vi "HDF5_Init_Validity_Refs.vi"(5 "HDF5 file ref":T2 format="%.0x", 9 "File Exists?":bool, 11 "error in":errorcluster) -> (4 "AlarmFileRefs":T1 {"Alarm_Source_dset" format="%.0x"; "Time_AlarmChange_dset" format="%.0x"; "Time_Valid_dset" format="%.0x"; "Alarm_Valid_dset" format="%.0x"; "Saturat_dset" format="%.0x"; "Group_ref" format="%.0x"; "Weath_Valid_dset" format="%.0x"; "Disdr_Valid_dset" format="%.0x"}, 15 "error out":errorcluster)   [LabVIEW 2018]
doc: "Set up the HDF5 data structure and initialize the references for the Noise1, Noise2, Noise3, and Noise4 Datasets (tables).\n\nData structure:\nNoise1 (Dataset) - 1024 element Double array (waveform) \nNoise2 (Dataset) - 1024 element Double array (waveform) \nNoise3 (Dataset) - 1024 element Double array (waveform) \nNoise4 (Dataset) - 1024 element Double array (waveform)"
uses:
  <vilib>/addons/h5labview2/base/hid_t.ctl
  HDF5_Validty_refs.ctl
  <vilib>/addons/h5labview2/base/lib_path.vi
  <vilib>/addons/h5labview2/base/H5Equery.vi
  lib_path_mod_20200519.vi
  <vilib>/addons/h5labview2/attrib/H5Awrite.llb/H5Awrite.xnode
  <vilib>/addons/h5labview2/group/H5G.lvlib
  <vilib>/addons/h5labview2/dataset/H5D.lvlib
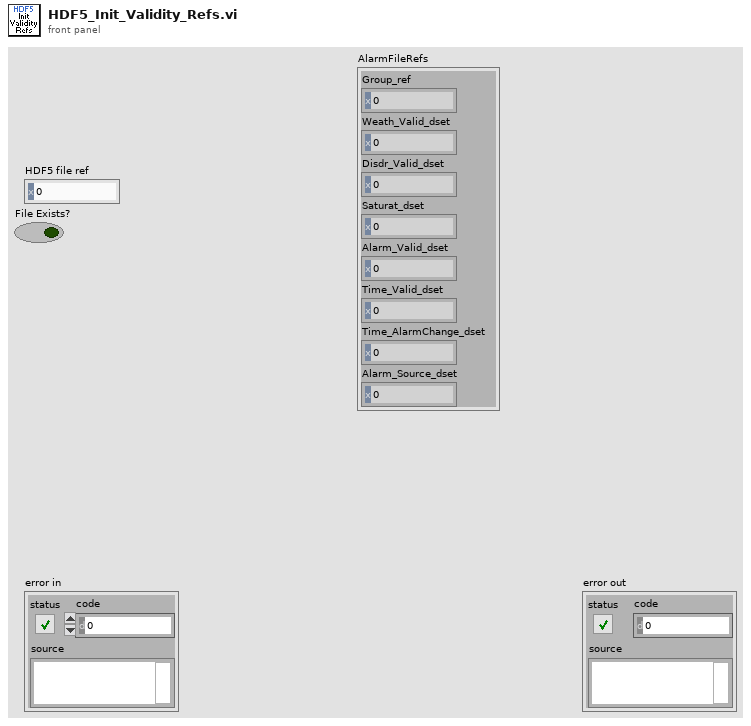
[diagram p1: front panel]
types:
  T1 = typedef "HDF5_Validty_refs.ctl" = cluster{"Group_ref":T2, "Weath_Valid_dset":T2, "Disdr_Valid_dset":T2, "Saturat_dset":T2, "Alarm_Valid_dset":T2, "Time_Valid_dset":T2, "Time_AlarmChange_dset":T2, "Alarm_Source_dset":T2}
  T2 = typedef "hid_t.ctl" = i32
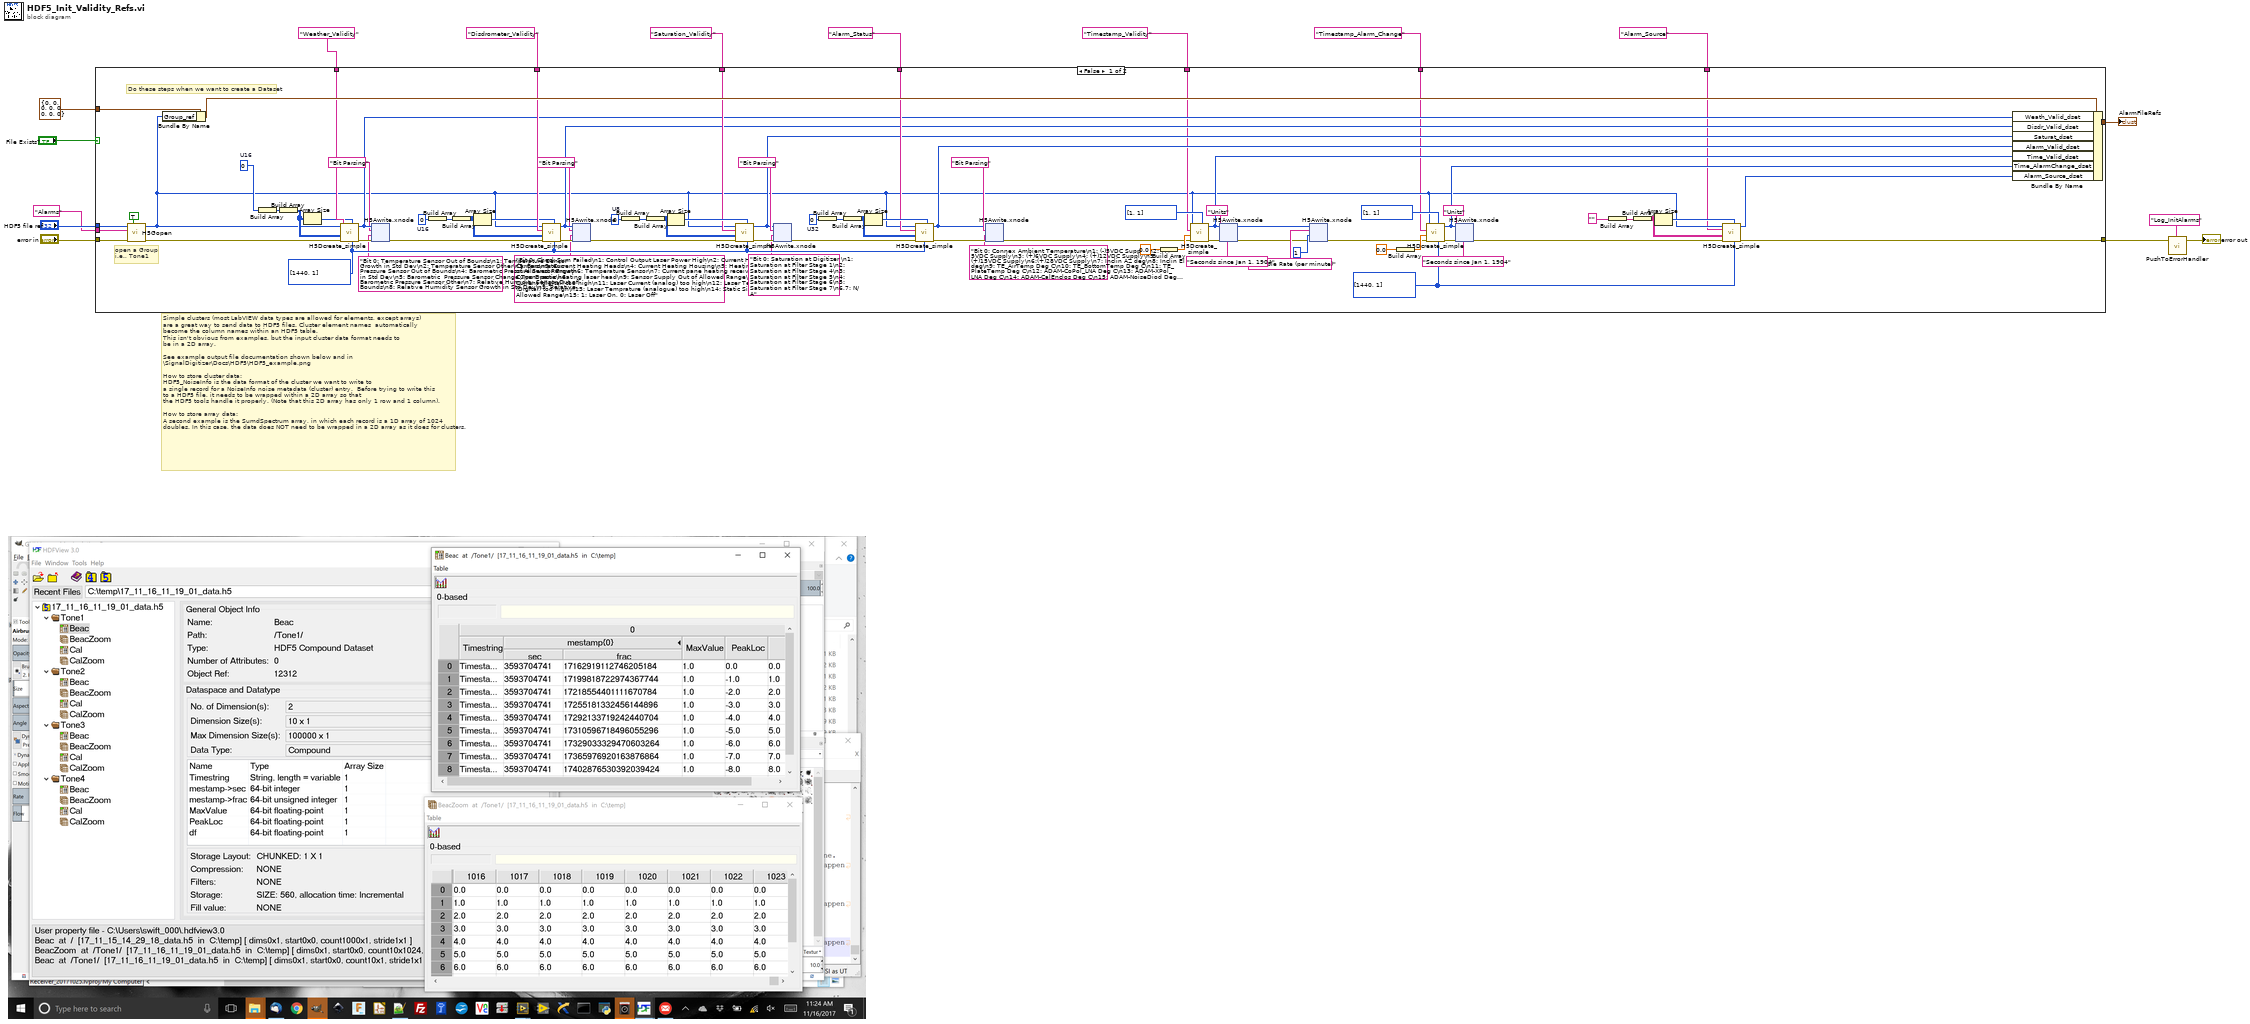
[diagram p0: block diagram]
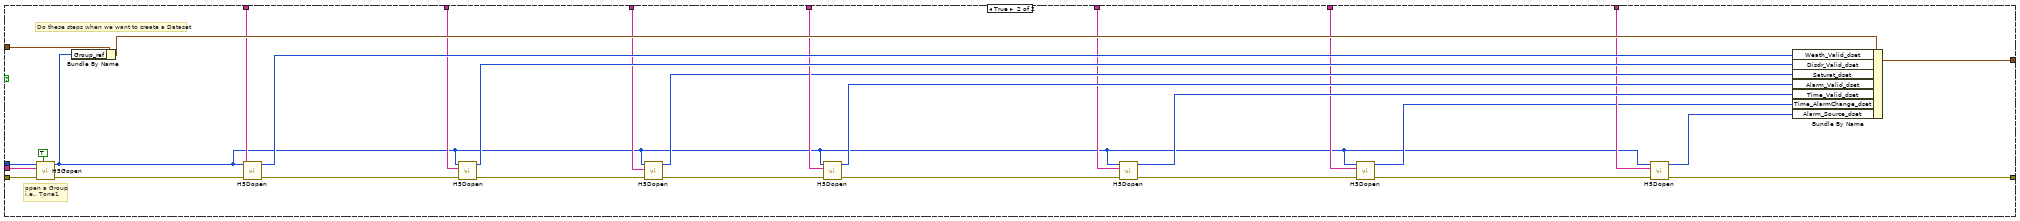
[diagram p2: hidden frame]
diagram:
  # "Simple clusters (most LabVIEW data types are allowed for elements, except arrays) \nare a great way to send data to HDF5 files. Cluster element names  automatically\nbecome the column names within an HDF5 table.\nThis isn't obvious from examples, but the input cluster data format needs to \nbe in a 2D array.\n\nSee example output file documentation shown below and in\n\\SignalDigitizer\\Docs\\HDF5\\HDF5_example.png\n\nHow to store cluster data:\nHDF5_NoiseInfo is the data format of the cluster we want to write to \na single record for a NoiseInfo noise metadata (cluster) entry.  Before trying to write this \nto a HDF5 file, it needs to be wrapped within a 2D array so that \nthe HDF5 tools handle it properly. (Note that this 2D array has only 1 row and 1 column).\n\nHow to store array data:\nA second example is the SumdSpectrum array, in which each record is a 1D array of 1024 \ndoubles. In this case, the data does NOT need to be wrapped in a 2D array as it does for clusters."
  n1 = case shown="False" "File Exists?" {
    tunnel: "error in" -> [w96 w259]
    tunnel: "HDF5 file ref" -> [w95 w258]
    tunnel: [w28 w235] -> w8
    tunnel: "Weather_Validity" ("string") -> [w89 w253]
    tunnel: "Disdrometer_Validity" ("string") -> [w88 w252]
    tunnel: T1 {"Group_ref"=0, "Weath_Valid_dset"=0, "Disdr_Valid_dset"=0, "Saturat_dset"=0, "Alarm_Valid_dset"=0, "Time_Valid_dset"=0, "Time_AlarmChange_dset"=0, "Alarm_Source_dset"=0} ("Cluster") -> [w85 w250]
    tunnel: "Alarms" ("name") -> [w84 w248]
    tunnel: [w83 w247] -> w10
    tunnel: "Saturation_Validity" ("string") -> [w74 w244]
    tunnel: "Alarm_Status" ("string") -> [w69 w243]
    tunnel: "Timestamp_Validity" ("string") -> [w37 w239]
    tunnel: "Timestamp_Alarm_Change" ("string") -> [w18 w234]
    tunnel: "Alarm_Source" ("string") -> [w17 w233]
    frame False {
      w22 = u64[] [1440, 1] ("max size")
      w70 = u32 0  # U32
      w78 = u8 0  # U8
      w79 = u16 0  # U16
      w80 = u16 0  # U16
      w68 = u64[] [1440, 1] ("max size")
      # "Do these steps when we want to create a Dataset"
      # "open a Group\ni.e., Tone1"
      n2 = call <vilib>:"H5Gopen.vi"("create? (F)"=TRUE, "error in (no error)"=w96, "name"=w84, "ref in"=w95) -> ("error out"=w91:errorcluster, "group out"=w24:T2)  [unwired: 6 in]
      n3 = Bundle By Name(cluster=w85, "Group_ref"=w24) -> (w90:T1)
      n4 = Build Array(w80) -> (w94:u16[])
      n5 = Build Array(w94) -> (w93:u16[][])
      n6 = Array Size(array=w93) -> (size(s)=w87:i32[])
      n7 = call <vilib>:"H5Dcreate_simple.vi"("max size"=w68, "chunk size"=w87, "error in (no error)"=w91, "type in"=w93, "name"=w89, "ref in"=w24) -> ("error out"=w67:errorcluster, "dset out"=w65:T2)  [unwired: 4 in]
      n8 = xnode "H5Awrite.xnode"("error in (no error)"=w67, "data"="Bit 0: Temperature Sensor Out of Bounds\n1: Temperature Sensor Growth in Std Dev\n2: Temperature Sensor Other\n3: Barometeric Pressure Sensor Out of Bounds\n4: Barometric Pressure Sensor Growth in Std Dev\n5: Barometric  Pressure Sensor Change Too Drastic\n6: Barometric Pressure Sensor Other\n7: Relative Humidity Sensor Out of Bounds\n8: Relative Humidity Sensor Growth in Std Dev\n9: Relative Humidity Sensor Other\n10: Wind Monitor Speed Out of Bounds\n11: Wind Monitor Direction Out of Bounds\n12: Rain Bucket Out of Bounds, too high\n13: Rain Bucket Not Reporting Precipitation Indicated by Disdrometer\n14: Disdrometer not reporting Precipitation Indicated By Rain Bucket\n15: Undefined", "attrib name"="Bit Parsing" ("object name"), "ref in"=w65) -> ("error out"=w66:errorcluster)  [unwired: 3 in, 2 out]
      n9 = Build Array(w79) -> (w82:u16[])
      n10 = Build Array(w82) -> (w81:u16[][])
      n11 = Array Size(array=w81) -> (size(s)=w86:i32[])
      n12 = call <vilib>:"H5Dcreate_simple.vi"("max size"=w68, "chunk size"=w86, "error in (no error)"=w66, "type in"=w81, "name"=w88, "ref in"=w24) -> ("error out"=w60:errorcluster, "dset out"=w62:T2)  [unwired: 4 in]
      n13 = xnode "H5Awrite.xnode"("error in (no error)"=w60, "data"="Bit 0: Check Sum Failed\n1: Control Output Laser Power High\n2: Current Heating Carriers\n3: Current Heating Heads\n4: Current Heating Housing\n5: Heating Supply Out of Allowed Range\n6: Temperature Sensor\n7: Current pane heating receiver head\n8: Current pane heating laser head\n9: Sensor Supply Out of Allowed Range\n10: Laser Current (digital) too high\n11: Laser Current (analog) too high\n12: Laser Temperature (Digital) too high\n13: Laser Temprature (analogue) too high\n14: Static Signal Out of Allowed Range\n15: 1: Laser On, 0: Laser Off" ("type name (default)"), "attrib name"="Bit Parsing" ("object name"), "ref in"=w62) -> ("error out"=w57:errorcluster)  [unwired: 3 in, 2 out]
      n14 = Build Array(w78) -> (w76:u8[])
      n15 = Build Array(w76) -> (w77:u8[][])
      n16 = Array Size(array=w77) -> (size(s)=w75:i32[])
      n17 = call <vilib>:"H5Dcreate_simple.vi"("max size"=w68, "chunk size"=w75, "error in (no error)"=w57, "type in"=w77, "name"=w74, "ref in"=w24) -> ("error out"=w58:errorcluster, "dset out"=w53:T2)  [unwired: 4 in]
      n18 = xnode "H5Awrite.xnode"("error in (no error)"=w58, "data"="Bit 0: Saturation at Digitizer \n1: Saturation at Filter Stage 1\n2: Saturation at Filter Stage 4\n3: Saturation at Filter Stage 5\n4: Saturation at Filter Stage 6\n5: Saturation at Filter Stage 7\n6,7: N/A" ("type name (default)"), "attrib name"="Bit Parsing" ("object name"), "ref in"=w53) -> ("error out"=w54:errorcluster)  [unwired: 3 in, 2 out]
      n19 = Build Array(w70) -> (w72:u32[])
      n20 = Build Array(w72) -> (w71:u32[][])
      n21 = Array Size(array=w71) -> (size(s)=w73:i32[])
      n22 = call <vilib>:"H5Dcreate_simple.vi"("max size"=w68, "chunk size"=w73, "error in (no error)"=w54, "type in"=w71, "name"=w69, "ref in"=w24) -> ("error out"=w55:errorcluster, "dset out"=w52:T2)  [unwired: 4 in]
      n23 = xnode "H5Awrite.xnode"("error in (no error)"=w55, "data"="Bit 0: Connex Ambient Temperature\n1: (-)5VDC Supply\n2: (+) 5VDC Supply\n3: (+)6VDC Supply\n4: (+)12VDC Supply\n5: (+)15VDC Supply\n6:(+)28VDC Supply\n7: Inclin AZ deg\n8: Inclin El deg\n9: TE_AirTemp Deg C\n10: TE_BottomTemp Deg C\n11: TE_PlateTemp Deg C\n12: ADAM-CoPol_LNA Deg C\n13: ADAM-XPol_LNA Deg C\n14: ADAM-CalEnclos Deg C\n15: ADAM-NoiseDiod Deg C\n16: 72Co_Beac_Freq MHz\n17: 72Co_Cal_Freq MHz\n18: 72Co_CalTonePower_dBM\n19: 72X_CalTonePower_dBM\n20: 84Co_Beac_Freq MHz\n21: 84Co_Cal_Freq MHz\n22: 84Co_CalTonePower_dBM\n23: 84X_CalTonePower_dBM\n24: 72Co_Beac_SNR<20 for 6hr\n25: 84Co_Beac_SNR<20 for 6 hr\n26: 72 GHz PLL Lock Status\n27: 84 GHz PLL Lock Status\n28-31: N/A" ("type name (default)"), "attrib name"="Bit Parsing" ("object name"), "ref in"=w52) -> ("error out"=w39:errorcluster)  [unwired: 3 in, 2 out]
      n24 = Build Array(0.0 ("Timestamp")) -> (w45:dbl[])
      n25 = call <vilib>:"H5Dcreate_simple.vi"("chunk size"=u64[] [1, 1], "error in (no error)"=w39, "type in"=w45, "name"=w37, "ref in"=w24) -> ("error out"=w48:errorcluster, "dset out"=w38:T2)  [unwired: 5 in]
      n26 = xnode "H5Awrite.xnode"("error in (no error)"=w48, "data"="Seconds since Jan 1, 1904", "attrib name"="Units", "ref in"=w38) -> ("error out"=w41:errorcluster, "ref out"=w40:i32)  [unwired: 3 in, 1 out]
      n27 = xnode "H5Awrite.xnode"("error in (no error)"=w41, "data"=u32 1, "attrib name"="Sample Rate (per minute)", "ref in"=w40) -> ("error out"=w23:errorcluster)  [unwired: 3 in, 2 out]
      n28 = Build Array(0.0 ("Timestamp")) -> (w33:dbl[])
      n29 = call <vilib>:"H5Dcreate_simple.vi"("max size"=w22, "chunk size"=u64[] [1, 1], "error in (no error)"=w23, "type in"=w33, "name"=w18, "ref in"=w24) -> ("error out"=w30:errorcluster, "dset out"=w29:T2)  [unwired: 4 in]
      n30 = xnode "H5Awrite.xnode"("error in (no error)"=w30, "data"="Seconds since Jan 1, 1904", "attrib name"="Units", "ref in"=w29) -> ("error out"=w20:errorcluster)  [unwired: 3 in, 2 out]
      n31 = Build Array("") -> (w26:string[])
      n32 = Build Array(w26) -> (w25:string[][])
      n33 = Array Size(array=w25) -> (size(s)=w27:i32[])
      n34 = call <vilib>:"H5Dcreate_simple.vi"("max size"=w22, "chunk size"=w27, "error in (no error)"=w20, "type in"=w25, "name"=w17, "ref in"=w24) -> ("error out"=w28:errorcluster, "dset out"=w21:T2)  [unwired: 4 in]
      n35 = Bundle By Name(cluster=w90, "Weath_Valid_dset"=w65, "Disdr_Valid_dset"=w62, "Saturat_dset"=w53, "Alarm_Valid_dset"=w52, "Time_Valid_dset"=w38, "Time_AlarmChange_dset"=w29, "Alarm_Source_dset"=w21) -> (w83:T1)
    }
    frame True {
      # "Do these steps when we want to create a Dataset"
      # "open a Group\ni.e., Tone1"
      n36 = call <vilib>:"H5Gopen.vi"("create? (F)"=TRUE, "error in (no error)"=w259, "name"=w248, "ref in"=w258) -> ("error out"=w256:errorcluster, "group out"=w230:T2)  [unwired: 6 in]
      n37 = Bundle By Name(cluster=w250, "Group_ref"=w230) -> (w255:T1)
      n38 = call <vilib>:"H5Dopen.vi"("error in (no error)"=w256, "name"=w253, "loc in"=w230) -> ("error out"=w249:errorcluster, "dset out"=w254:T2)  [unwired: 7 in]
      n39 = call <vilib>:"H5Dopen.vi"("error in (no error)"=w249, "name"=w252, "loc in"=w230) -> ("error out"=w246:errorcluster, "dset out"=w251:T2)  [unwired: 7 in]
      n40 = call <vilib>:"H5Dopen.vi"("error in (no error)"=w246, "name"=w244, "loc in"=w230) -> ("error out"=w245:errorcluster, "dset out"=w242:T2)  [unwired: 7 in]
      n41 = call <vilib>:"H5Dopen.vi"("error in (no error)"=w245, "name"=w243, "loc in"=w230) -> ("error out"=w240:errorcluster, "dset out"=w241:T2)  [unwired: 7 in]
      n42 = call <vilib>:"H5Dopen.vi"("error in (no error)"=w240, "name"=w239, "loc in"=w230) -> ("error out"=w236:errorcluster, "dset out"=w238:T2)  [unwired: 7 in]
      n43 = call <vilib>:"H5Dopen.vi"("error in (no error)"=w236, "name"=w234, "loc in"=w230) -> ("error out"=w237:errorcluster, "dset out"=w232:T2)  [unwired: 7 in]
      n44 = call <vilib>:"H5Dopen.vi"("error in (no error)"=w237, "name"=w233, "loc in"=w230) -> ("error out"=w235:errorcluster, "dset out"=w231:T2)  [unwired: 7 in]
      n45 = Bundle By Name(cluster=w255, "Weath_Valid_dset"=w254, "Disdr_Valid_dset"=w251, "Saturat_dset"=w242, "Alarm_Valid_dset"=w241, "Time_Valid_dset"=w238, "Time_AlarmChange_dset"=w232, "Alarm_Source_dset"=w231) -> (w247:T1)
    }
  }
  "AlarmFileRefs" <- w10
  n46 = call "PushToErrorHandler.vi"("ErrorIn"=w8, "ErrorLocation"="Log_InitAlarms") -> ("ErrorOut"=→"error out":errorcluster)  [unwired: 5 in]
